vi "Video livestream (TCP SERVER).vi"(1 "Quality":i32=750 min=0 max=1000, 2 "TCP/IP port":u16=80, 3 "VideoMode":u32, 4 "Interface name":T1="Travcam") -> (0 "Error Out":errorcluster)   [LabVIEW 2015]
doc: "This VI must be loaded when the camera server starts, and also in the list of exported VIs. This VI is not to run directly."
uses:
  <vilib>/userdefined/High Color/IMAQdx.ctl
  <vilib>/vision/driver/IMAQdx.llb/IMAQdx Camera Control Mode.ctl
  <vilib>/vision/driver/NI_Vision_Acquisition_Software.lvlib
  <resource>/objmgr/imaqdx.rc
panel:
  in  "Stop":bool
  out "Video":T2(plugin-control)
  # "PN 27/08/2015"
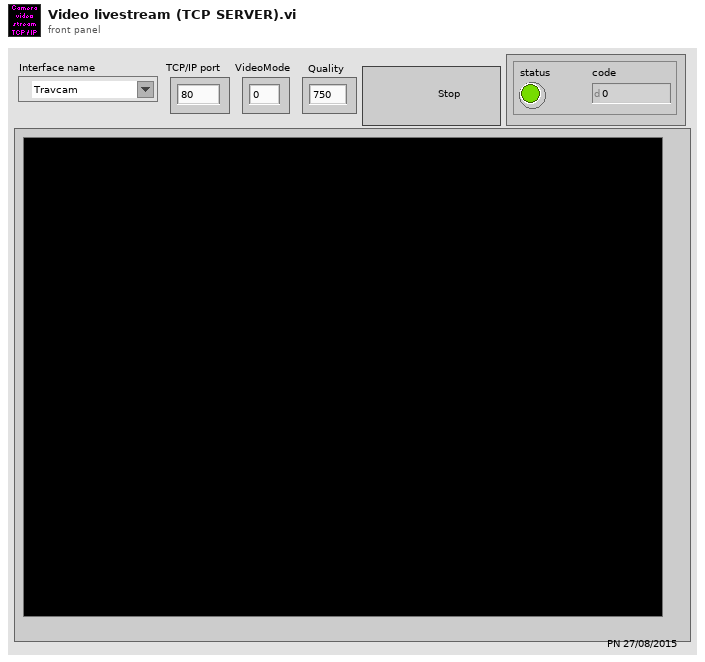
[diagram p1: front panel]
types:
  T1 = typedef "IMAQdx.ctl" = refnum<k21>
  T2 = typedef "IMAQ Image.ctl" = refnum<image>
  T3 = typedef "Image Type" = u32
  T4 = typedef "NI_Vision_Acquisition_Software.lvlib/IMAQdx Camera Control Mode.ctl" = enum32{"Controller", "Listener"}
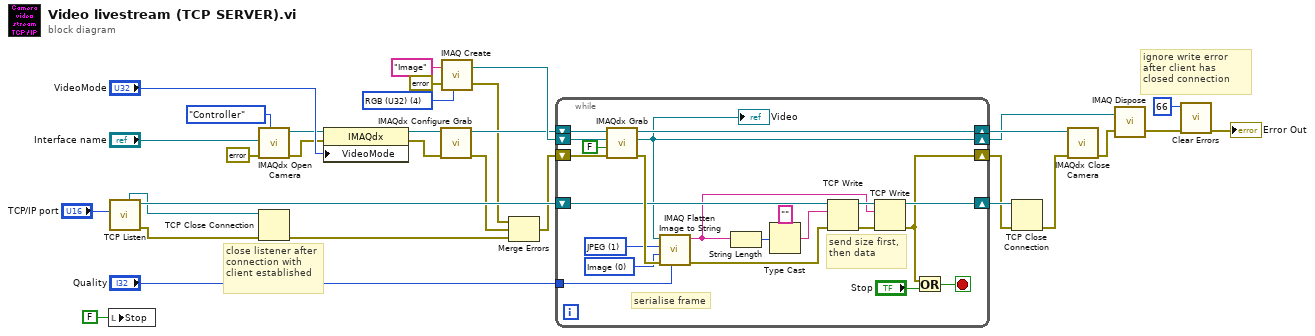
[diagram p0: block diagram]
diagram:
  w26 = T3 4 items=["Grayscale (U8)", "Grayscale (I16)", "Grayscale (SGL)", "Complex (CSG)", "RGB (U32)", "HSL (U32)", "RGB (U64)", "Grayscale (U16)"] ("Image Type")
  # "ignore write error after client has closed connection"
  # "close listener after connection with client established"
  n1 = local write "Stop"(FALSE ("Stop")) -> ()
  n2 = call <vilib>:"TCP Listen.vi"("port"="TCP/IP port") -> ("error out"=w10:errorcluster, "connection ID"=w30:refnum<k5>, "listener ID"=w11:refnum<k5>)  [unwired: 6 in, 2 out]
  n3 = call <vilib>:"IMAQdx Open Camera.vi"("Camera Control Mode"=IMAQdx_Camera_Control_Mode."Controller", "error in"=errorcluster {"status"=FALSE, "code"=0, "source"=""}, "Session In"="Interface name") -> ("error out"=w19:errorcluster, "Session Out"=w17:T1)  [unwired: 7 in]
  n4 = TCP Close Connection(connection ID=w11, error in (no error)=w10) -> (error out=w9:errorcluster)  [unwired: 1 in, 1 out]
  n5 = property class="IMAQdx"(reference=w17, error in=w19, "VideoMode"="VideoMode") -> (reference out=w20:T1, error out=w18:errorcluster)
  n6 = call <vilib>:"IMAQdx Configure Grab.vi"("error in"=w18, "Session In"=w20) -> ("error out"=w14:errorcluster, "Session Out"=w21:T1)  [unwired: 8 in]
  n7 = call "IMAQ Create"("Image Name"="Image", "Image Type"=w26, "error in (no error)"=errorcluster {"status"=FALSE, "code"=0, "source"=""} ("error in")) -> ("New Image"=w25:T2, "error out"=w2:errorcluster)  [unwired: 2 in]
  n8 = Merge Errors(w2, w14, w9) -> (w13:errorcluster)
  n9 = while {
    shift-right: [w52] -> w24
    shift-left: w21 -> [w54]
    shift-right: [w34] -> w23
    shift-left: w25 -> [w53]
    shift-right: [w36] -> w7
    shift-left: w13 -> [w51]
    shift-right: [w37] -> w12
    shift-left: w30 -> [w42]
    tunnel: "Quality" -> [w33]
    stop <- w49 stop-if-true
    w45 = 1 items=["None", "JPEG", "PACKED BINARY"] ("Compression (None)")
    w46 = 0 items=["Image", "Image and Vision Info", "Reference to Image"] ("Type of Flatten (Image and Vision Info)")
    # "serialise frame"
    # "send size first, then data"
    n10 = call <vilib>:"IMAQdx Grab.vi"("error in"=w51, "Wait for Next Buffer? (Yes)"=FALSE, "Image In"=w53, "Session In"=w54) -> ("error out"=w47:errorcluster, "Image Out"=w34:T2, "Session Out"=w52:T1)  [unwired: 4 in, 1 out]
    "Video" <- w34
    n11 = call "IMAQ Flatten Image to String"("Quality (750)"=w33, "error in (no error)"=w47, "Type of Flatten (Image and Vision Info)"=w46, "Compression (None)"=w45, "Image"=w34) -> ("error out"=w40:errorcluster, "Data String"=w35:string)  [unwired: 5 in]
    n12 = String Length(string=w35) -> (length=w44:i32)
    n13 = Type Cast(type="", x=w44) -> (*(type *) &x=w41:string)
    n14 = TCP Write(connection ID=w42, data in=w41, error in (no error)=w40) -> (connection ID out=w38:refnum<k5>, error out=w39:errorcluster)  [unwired: 1 in, 1 out]
    n15 = TCP Write(connection ID=w38, data in=w35, error in (no error)=w39) -> (connection ID out=w37:refnum<k5>, error out=w36:errorcluster)  [unwired: 1 in, 1 out]
    n16 = Or(x=w36, y="Stop") -> (x .or. y?=w49:bool)
  }
  n17 = TCP Close Connection(connection ID=w12, error in (no error)=w7) -> (error out=w6:errorcluster)  [unwired: 1 in, 1 out]
  n18 = call <vilib>:"IMAQdx Close Camera.vi"("error in"=w6, "Session In"=w24) -> ("error out"=w22:errorcluster)  [unwired: 9 in]
  n19 = call "IMAQ Dispose"("Image"=w23, "error in (no error)"=w22) -> ("error out"=w3:errorcluster)  [unwired: 4 in]
  n20 = call <vilib>:"Clear Errors.vi"("error in (no error)"=w3, "specific error code to clear (0: all)"=66) -> ("error out"=→"Error Out":errorcluster)  [unwired: 4 in, 1 out]
